vi "Excel Find and Replace (str).vi"(0 "report in":refnum<class "NI_report.lvclass">, 5 "searched string":string, 7 "replacement":string, 11 "error in (no error)":errorcluster) -> (4 "report out":refnum<class "NI_report.lvclass">, 8 "found?":bool, 15 "error out":errorcluster)   [LabVIEW 2017, in "NI_Excel.lvclass"]
doc: "Searches the occurrences of <B>searched string</B> and replaces them with a new string or numeric value. The data type you wire to the <B>replacement</B> input determines the polymorphic instance to use."
uses:
  <vilib>/Utility/NIReport.llb/Excel/NI_Excel.lvclass
  <vilib>/Utility/NIReport.llb/NI_report.lvclass
  C:/Program Files (x86)/National Instruments/LabVIEW 2017/vi.lib/Utility/NIReport.llb/NI_report.lvclass
  <vilib>/Utility/NIReport.llb/Excel/NI_Excel.lvclass/NI_Excel.ctl
  <vilib>/Utility/NIReport.llb/NI_ReportGenerationCore.lvlib
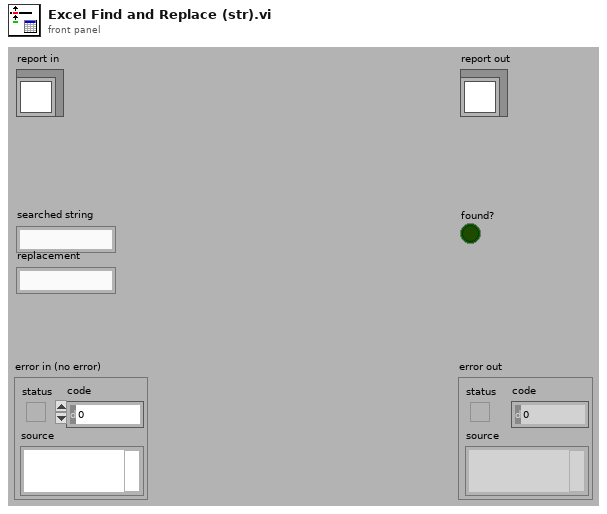
[diagram p1: front panel]
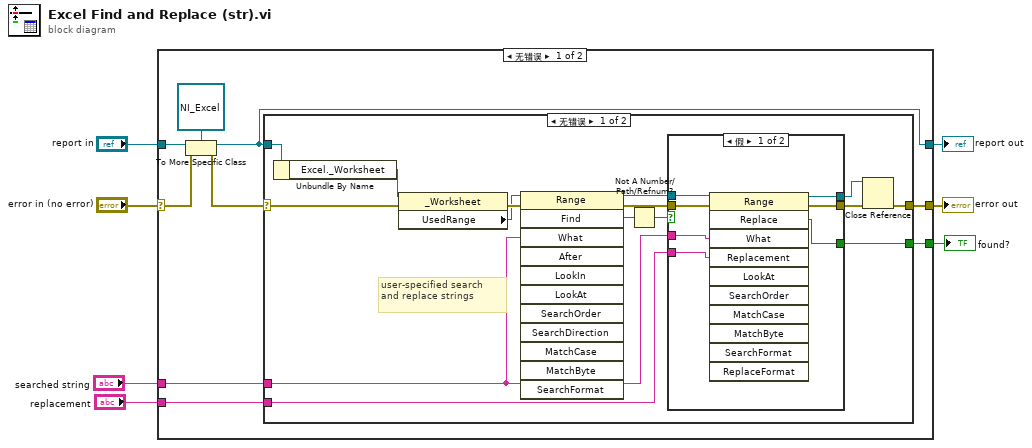
[diagram p0: block diagram]
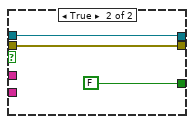
[diagram p2: hidden frame]
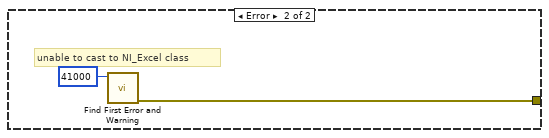
[diagram p3: hidden frame]
diagram:
  n1 = case shown="无错误" "error in (no error)" {
    selector: "error in (no error)" -> [w9 w45]
    tunnel: [w16 w45] -> w6
    tunnel: [w11 w44] -> w4
    tunnel: "report in" -> [w12 w44]
    tunnel: "replacement" -> [w15 _]
    tunnel: "searched string" -> [w14 _]
    tunnel: [w8 _] -> w1
    frame No Error {
      n2 = To More Specific Class(target class=refnum<class "NI_Excel.lvclass"> refnum ("report in"), reference=w12, error in=w9) -> (specific class reference=w11:refnum<class "NI_Excel.lvclass">, error out=w10:errorcluster)
      n3 = case shown="无错误" w10 {
        selector: w10 -> [w28 _]
        tunnel: [w30 w42] -> w16
        tunnel: w15 -> [w22 _]
        tunnel: w14 -> [w23 _]
        tunnel: w11 -> [w29 _]
        tunnel: [w17 _] -> w8
        frame No Error {
          # "user-specified search\nand replace strings"
          n4 = Unbundle By Name(w29) -> ("Excel._Worksheet"=w31:refnum<k7>)
          n5 = property class="_Worksheet"(reference=w31, error in=w28) -> (error out=w27:errorcluster, "UsedRange"=w26:refnum<k7>)  [unwired: 1 out]
          n6 = invoke class="Range" method="Find"(reference=w26, error in=w27, "What"=w23) -> (reference out=w21:refnum<k7>, error out=w20:errorcluster, "Find"=w25:refnum<k7>)  [unwired: 9 in, 9 out]
          n7 = Not A Number/Path/Refnum?(number/path/refnum=w25) -> (NaN/Path/Refnum?=w24:bool)
          n8 = case shown="假" w24 {
            tunnel: w23 -> [w38 _]
            tunnel: w22 -> [w37 _]
            tunnel: w21 -> [w36 w41]
            tunnel: [w35 w41] -> w18
            tunnel: w20 -> [w34 w40]
            tunnel: [w33 w40] -> w19
            tunnel: [w32 FALSE ("found?")] -> w17
            frame False {
              n9 = invoke class="Range" method="Replace"(reference=w36, error in=w34, "What"=w38, "Replacement"=w37) -> (reference out=w35:refnum<k7>, error out=w33:errorcluster, "Replace"=w32:bool)  [unwired: 7 in, 8 out]
            }
            frame True {
            }
          }
          n10 = Close Reference(reference=w18, error in (no error)=w19) -> (error out=w30:errorcluster)
        }
        frame Error {
          # "unable to cast to NI_Excel class"
          n11 = call <vilib>:"Find First Error and Warning.vi"("error code"=41000) -> ("error out"=w42:errorcluster)  [unwired: 2 in, 4 out]
        }
      }
    }
    frame Error {
    }
  }
  "error out" <- w6
  "report out" <- w4
  "found?" <- w1
